vi "target - Copy.vi"   [LabVIEW 2020]
uses:
  <vilib>/rvi/interface/RandomDataEmulation/niFpgaRandomDataHandleErrors.vi
  <vilib>/rvi/DataTransferAndStorage/Container/XNode/niFpgaContainer.xnode
  <vilib>/rvi/interface/RandomDataEmulation/nirviRandomDataFpgaReadWriteTemplate.vi
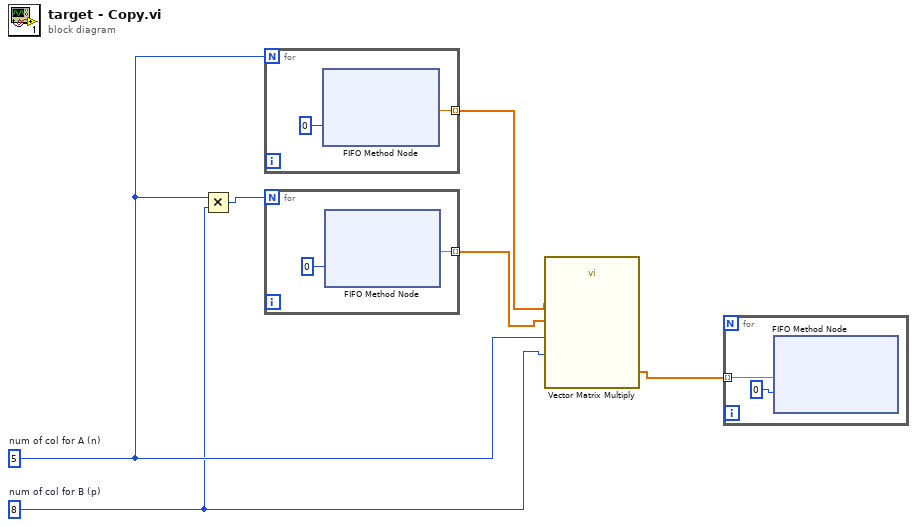
[diagram p0: block diagram]
diagram:
  w1 = 8  # num of col for B (p)
  w2 = 5  # num of col for A (n)
  n1 = Multiply(x=w2, y=w1) -> (x*y=w3:i32)
  n2 = for {
    N: w2 -> [_]
    tunnel: [w8] -> w6 mode=indexing
    n3 = xnode ("FIFO Method Node")("Timeout"=0) -> ("Element"=w8:sgl)  [unwired: 1 in, 2 out]
  }
  n4 = for {
    N: w3 -> [_]
    tunnel: [w9] -> w5 mode=indexing
    n5 = xnode ("FIFO Method Node")("Timeout"=0) -> ("Element"=w9:sgl)  [unwired: 1 in, 2 out]
  }
  n6 = call "Vector Matrix Multiply.vi"("p"=w1, "n"=w2, "B"=w5, "A"=w6) -> ("C"=w4:sgl[])
  n7 = for {
    tunnel: w4 -> [w12] mode=indexing
    n8 = xnode ("FIFO Method Node")("Element"=w12, "Timeout"=0) -> ()  [unwired: 1 in, 2 out]
  }
